vi "Teleop Drive Dispatch.vi"(9 "Button Values":bool[](array[boolean]), 10 "array":dbl[](array[numeric])) -> ()   [LabVIEW 2017]
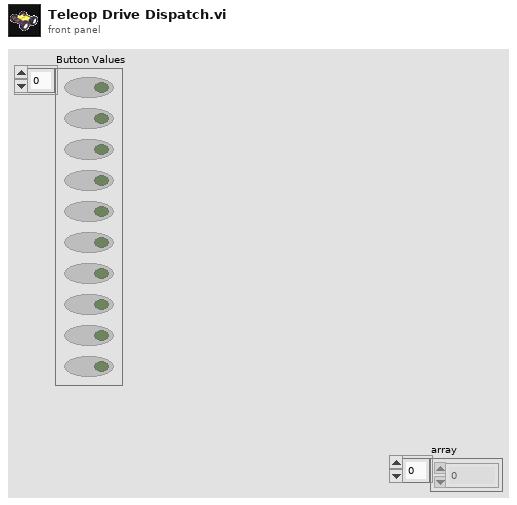
[diagram p1: front panel]
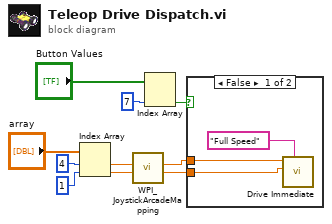
[diagram p0: block diagram]
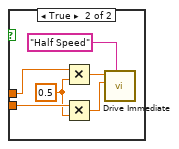
[diagram p2: hidden frame]
diagram:
  n1 = Index Array(array="array", index #1=4 ("index"), index #2=1 ("index")) -> (element #1=w10:dbl, element #2=w9:dbl)
  n2 = call <vilib>:"WPI_JoystickArcadeMapping.vi"("Y axis value"=w9, "X axis value"=w10) -> ("Right Motor Value"=w7:dbl, "Left Motor Value"=w6:dbl)  [unwired: 8 in]
  n3 = Index Array(array="Button Values", index #2=7 ("index")) -> (element #2=w3:bool)  [unwired: 1 in, 1 out]
  n4 = case shown="False" w3 {
    tunnel: w7 -> [w12 w18]
    tunnel: w6 -> [w11 w19]
    frame False {
      n5 = call "Drive Immediate.vi"("Description"="Full Speed", "Right Setpoint"=w12, "Left Setpoint"=w11) -> ()  [unwired: 8 in, 1 out]
    }
    frame True {
      w17 = 0.5
      n6 = Multiply(x=w19, y=w17) -> (x*y=w16:dbl)
      n7 = Multiply(x=w18, y=w17) -> (x*y=w15:dbl)
      n8 = call "Drive Immediate.vi"("Description"="Half Speed", "Right Setpoint"=w15, "Left Setpoint"=w16) -> ()  [unwired: 8 in, 1 out]
    }
  }
